vi "TestSekansiBaslat.vi"(10 "içecek":i64, 11 "queue in":refnum<queue>) -> ()   [LabVIEW 2021]
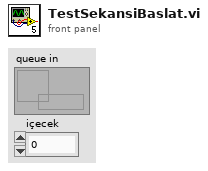
[diagram p1: front panel]
types:
  T1 = cluster{"element":string, "Message Data":variant}
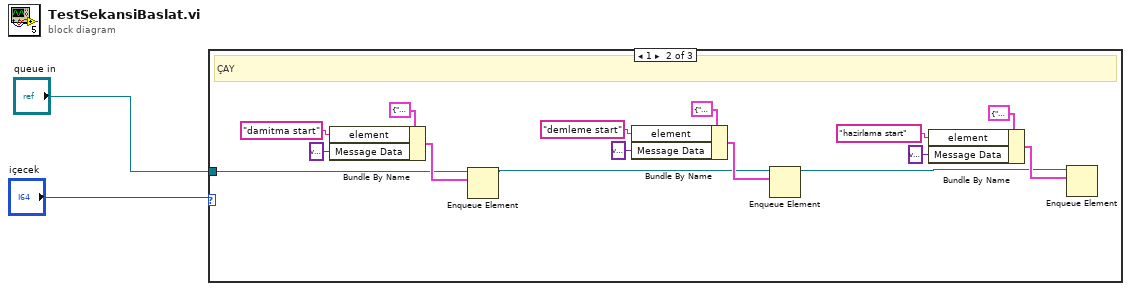
[diagram p0: block diagram]
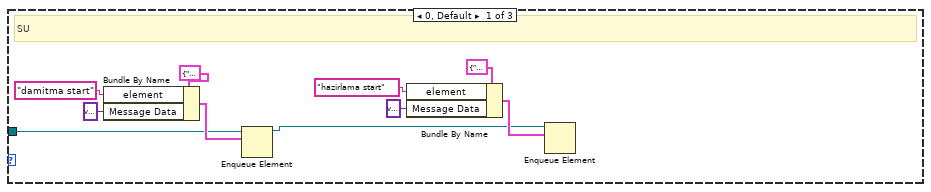
[diagram p2: hidden frame]
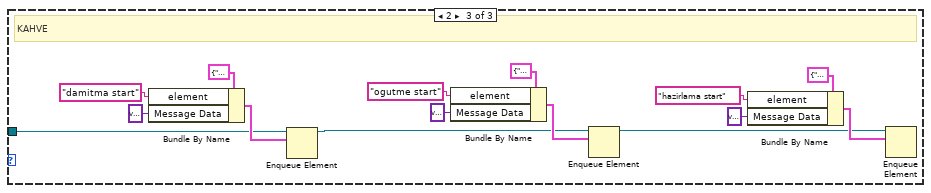
[diagram p3: hidden frame]
diagram:
  n1 = case shown="1" "içecek" {
    tunnel: "queue in" -> [w4 w15 w30]
    frame 0, Default {
      # "SU"
      n2 = Bundle By Name(cluster=T1 {"element"="", "Message Data"=variant}, "element"="damitma start", "Message Data"=variant) -> (w11:T1)
      n3 = Enqueue Element(queue=w4, element=w11) -> (queue out=w3:refnum<queue>)  [unwired: 2 in, 2 out]
      n4 = Bundle By Name(cluster=T1 {"element"="", "Message Data"=variant}, "element"="hazirlama start", "Message Data"=variant) -> (w12:T1)
      n5 = Enqueue Element(queue=w3, element=w12) -> ()  [unwired: 2 in, 3 out]
    }
    frame 1 {
      # "ÇAY"
      n6 = Bundle By Name(cluster=T1 {"element"="", "Message Data"=variant}, "element"="damitma start", "Message Data"=variant) -> (w24:T1)
      n7 = Enqueue Element(queue=w15, element=w24) -> (queue out=w14:refnum<queue>)  [unwired: 2 in, 2 out]
      n8 = Bundle By Name(cluster=T1 {"element"="", "Message Data"=variant}, "element"="demleme start", "Message Data"=variant) -> (w23:T1)
      n9 = Enqueue Element(queue=w14, element=w23) -> (queue out=w13:refnum<queue>)  [unwired: 2 in, 2 out]
      n10 = Bundle By Name(cluster=T1 {"element"="", "Message Data"=variant}, "element"="hazirlama start", "Message Data"=variant) -> (w16:T1)
      n11 = Enqueue Element(queue=w13, element=w16) -> ()  [unwired: 2 in, 3 out]
    }
    frame 2 {
      # "KAHVE"
      n12 = Bundle By Name(cluster=T1 {"element"="", "Message Data"=variant}, "element"="damitma start", "Message Data"=variant) -> (w39:T1)
      n13 = Enqueue Element(queue=w30, element=w39) -> (queue out=w29:refnum<queue>)  [unwired: 2 in, 2 out]
      n14 = Bundle By Name(cluster=T1 {"element"="", "Message Data"=variant}, "element"="ogutme start", "Message Data"=variant) -> (w38:T1)
      n15 = Enqueue Element(queue=w29, element=w38) -> (queue out=w28:refnum<queue>)  [unwired: 2 in, 2 out]
      n16 = Bundle By Name(cluster=T1 {"element"="", "Message Data"=variant}, "element"="hazirlama start", "Message Data"=variant) -> (w31:T1)
      n17 = Enqueue Element(queue=w28, element=w31) -> ()  [unwired: 2 in, 3 out]
    }
  }
